vi "_SetOneLibSO.vi"(6 "error in (no error)":errorcluster, 8 "Path":path, 9 "Set":bool) -> (0 "error out":errorcluster)   [LabVIEW 2014]
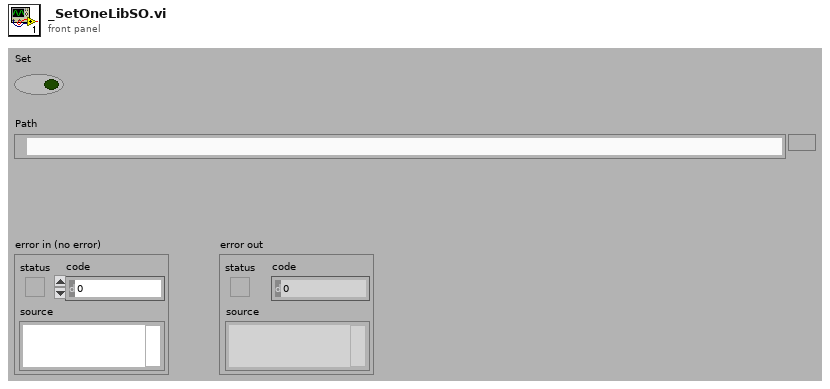
[diagram p1: front panel]
types:
  T1 = enum32{"invalid lock state", "Not Locked", "Locked (No Password)", "Password-protected"}
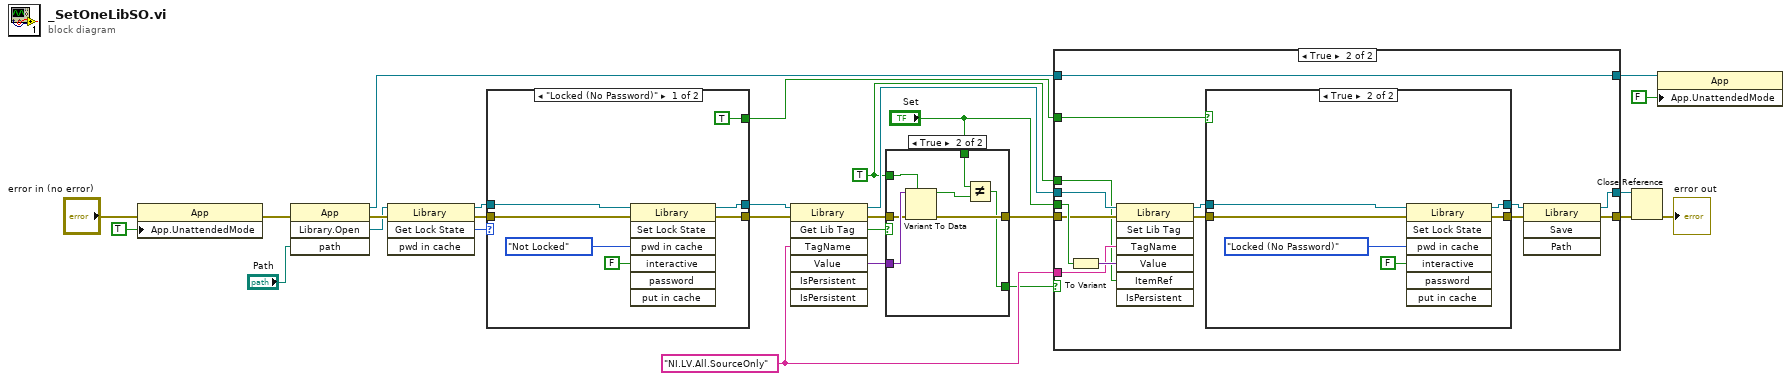
[diagram p0: block diagram]
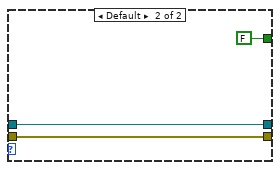
[diagram p2: hidden frame]
diagram:
  w24 = "NI.LV.All.SourceOnly" ("Tag Name")
  w7 = TRUE
  n1 = property class="App"(error in="error in (no error)", "App.UnattendedMode"=TRUE ("Application:Unattended Mode")) -> (error out=w27:errorcluster)  [unwired: 1 in, 1 out]
  n2 = invoke class="App" method="Library.Open"(error in=w27, "path"="Path") -> (reference out=w4:refnum<vi>, error out=w19:errorcluster, "Open Library"=w15:refnum<vi>)  [unwired: 2 in, 1 out]
  n3 = invoke class="Library" method="Get Lock State"(reference=w15, error in=w19) -> (reference out=w21:refnum<vi>, error out=w20:errorcluster, "Get Lock State"=w22:T1)  [unwired: 2 in, 1 out]
  n4 = case shown="\"Locked (No Password)\"" w22 {
    tunnel: w21 -> [w33 w37]
    tunnel: [w32 w37] -> w18
    tunnel: w20 -> [w31 w36]
    tunnel: [w30 w36] -> w14
    tunnel: [TRUE FALSE] -> w11
    frame "Locked (No Password)" {
      n5 = invoke class="Library" method="Set Lock State"(reference=w33, error in=w31, "pwd in cache"=T1."Not Locked" ("lock state"), "interactive"=FALSE) -> (reference out=w32:refnum<vi>, error out=w30:errorcluster)  [unwired: 3 in, 5 out]
    }
    frame Default {
    }
  }
  n6 = invoke class="Library" method="Get Lib Tag"(reference=w18, error in=w14, "TagName"=w24) -> (reference out=w17:refnum<vi>, error out=w16:errorcluster, "GetTag"=w23:bool, "Value"=w26:variant)  [unwired: 4 in, 3 out]
  n7 = case shown="True" w23 {
    tunnel: w26 -> [_ w46]
    tunnel: w16 -> [w39 w45]
    tunnel: [w39 w44] -> w25
    tunnel: w7 -> [w38 w43]
    tunnel: "Set" -> [_ w41]
    tunnel: [w38 w40] -> w1
    frame False {
    }
    frame True {
      n8 = Variant To Data(error in=w45, type=w43, Variant=w46) -> (data=w42:bool, error out=w44:errorcluster)
      n9 = Not Equal?(x=w41, y=w42) -> (x != y?=w40:bool)
    }
  }
  n10 = case shown="True" w1 {
    tunnel: [w48 w58] -> w13
    tunnel: [w49 w57] -> w12
    tunnel: "Set" -> [_ w62]
    tunnel: w25 -> [w49 w61]
    tunnel: w17 -> [w48 w60]
    tunnel: w24 -> [_ w59]
    tunnel: w11 -> [_ w52]
    tunnel: w7 -> [_ w51]
    tunnel: w4 -> [w47 w50]
    tunnel: [w47 w50] -> w5
    frame False {
    }
    frame True {
      n11 = To Variant(anything=w62) -> (Variant=w63:variant)
      n12 = invoke class="Library" method="Set Lib Tag"(reference=w60, error in=w61, "TagName"=w59, "Value"=w63, "ItemRef"=w51) -> (reference out=w56:refnum<vi>, error out=w55:errorcluster)  [unwired: 2 in, 5 out]
      n13 = case shown="True" w52 {
        tunnel: w56 -> [w65 w71]
        tunnel: w55 -> [w64 w70]
        tunnel: [w65 w69] -> w54
        tunnel: [w64 w68] -> w53
        frame False {
        }
        frame True {
          n14 = invoke class="Library" method="Set Lock State"(reference=w71, error in=w70, "pwd in cache"=T1."Locked (No Password)" ("lock state"), "interactive"=FALSE) -> (reference out=w69:refnum<vi>, error out=w68:errorcluster)  [unwired: 3 in, 5 out]
        }
      }
      n15 = invoke class="Library" method="Save"(reference=w54, error in=w53) -> (reference out=w58:refnum<vi>, error out=w57:errorcluster)  [unwired: 2 in, 2 out]
    }
  }
  n16 = Close Reference(reference=w13, error in (no error)=w12) -> (error out=→"error out":errorcluster)
  n17 = property class="App"(reference=w5, "App.UnattendedMode"=FALSE ("Application:Unattended Mode")) -> ()  [unwired: 1 in, 2 out]
